vi "Get Historic Data.vi"(0 "lvFinanceFunctionsHL in":refnum<class "lvFinanceFunctionsHL.lvclass">, 5 "Period":T2(ring), 7 "Interval":T1(ring), 11 "error in (no error)":errorcluster) -> (4 "lvFinanceFunctionsHL out":refnum<class "lvFinanceFunctionsHL.lvclass">, 6 "Historic Data":cluster{timestamp[], dbl[][]}, 15 "error out":errorcluster)   [LabVIEW 2020, in "lvFinanceFunctionsHL.lvclass"]
uses:
  lvFinanceFunctionsHL.lvclass
  lvFinanceFunctionsHL.lvclass/lvFinanceFunctionsHL.ctl
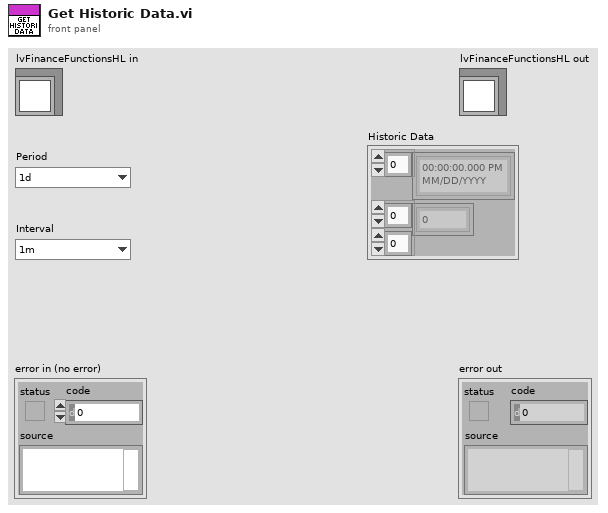
[diagram p1: front panel]
types:
  T1 = enum16{"1m", "2m", "5m", "15m", "30m", "60m", "90m", "1h", "1d", "5d", "1wk", "1mo", "3mo"}
  T2 = enum16{"1d", "5d", "1mo", "3mo", "6mo", "1y", "2y", "5y", "10y", "ytd", "max"}
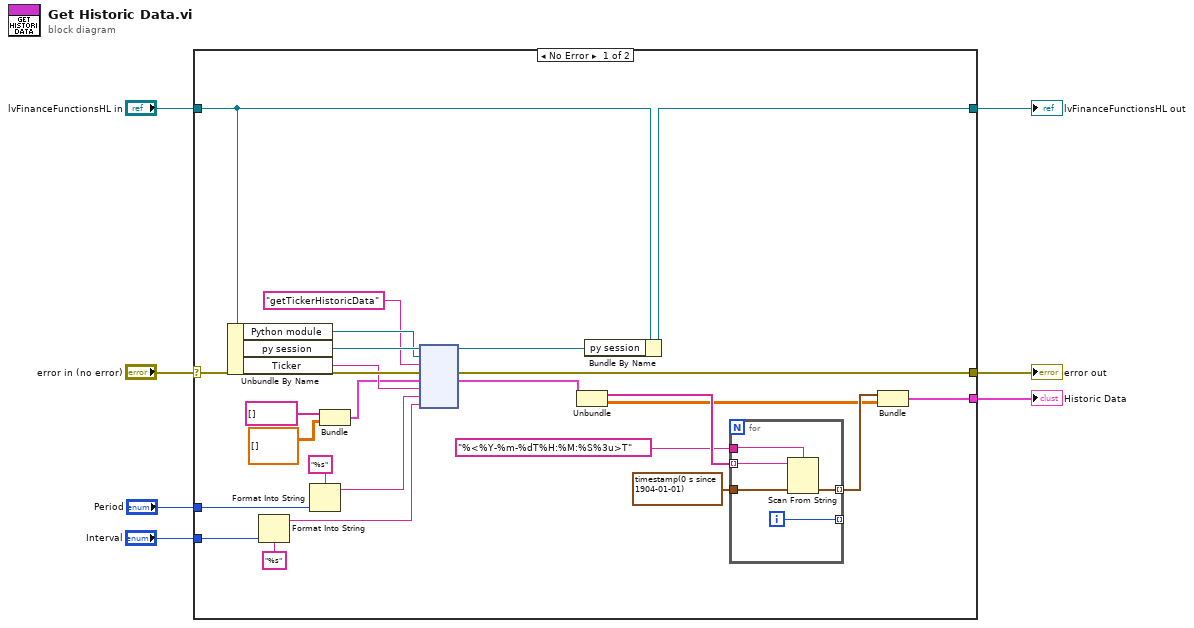
[diagram p0: block diagram]
diagram:
  n1 = case shown="No Error" "error in (no error)" {
    selector: "error in (no error)" -> [w28 w39]
    tunnel: [w27 w39] -> w6
    tunnel: [w30 w38] -> w4
    tunnel: "lvFinanceFunctionsHL in" -> [w29 w38]
    tunnel: [w14 _] -> w3
    tunnel: "Period" -> [w13 _]
    tunnel: "Interval" -> [w9 _]
    frame No Error {
      n2 = Unbundle By Name(w29) -> ("Python module"=w26:path, "py session"=w32:refnum<k35>, "Ticker"=w24:string)
      n3 = Format Into String(format string="%s", w9) -> (resulting string=w8:string)  [unwired: 2 in, 1 out]
      n4 = Format Into String(format string="%s", w13) -> (resulting string=w11:string)  [unwired: 2 in, 1 out]
      n5 = Bundle(string[] [], dbl[][] []) -> (w21:cluster{string[], dbl[][]})  [unwired: 1 in]
      n6 = node(w32, w26, "getTickerHistoricData" ("function name"), w28, w21, w24, w11, w8) -> (w31:refnum<k35>, w27:errorcluster, w17:cluster{string[], dbl[][]})  [unwired: 3 in, 2 out]
      n7 = Unbundle(w17) -> (w20:string[], w15:dbl[][])
      n8 = Bundle By Name(cluster=w29, "py session"=w31) -> (w30:refnum<class "lvFinanceFunctionsHL.lvclass">)
      n9 = for {
        tunnel: w20 -> [w37] mode=indexing
        tunnel: "%<%Y-%m-%dT%H:%M:%S%3u>T" ("format string") -> [w36]
        tunnel: timestamp(0 s since 1904-01-01) -> [w35]
        tunnel: [w34] -> w16 mode=indexing
        tunnel: [w33] -> _ mode=indexing
        i -> [w33]
        n10 = Scan From String(format string=w36, input string=w37, default 1=w35) -> (output 1=w34:timestamp)  [unwired: 2 in, 3 out]
      }
      n11 = Bundle(w16, w15) -> (w14:cluster{timestamp[], dbl[][]})  [unwired: 1 in]
    }
    frame Error {
    }
  }
  "error out" <- w6
  "lvFinanceFunctionsHL out" <- w4
  "Historic Data" <- w3
